vi "Process.vi"(8 "error in":errorcluster, 11 "XYStage.KIM101":refnum<class "XYStage.KIM101.lvclass">) -> (0 "error out":errorcluster, 3 "XYStage.KIM101 out":refnum<class "XYStage.KIM101.lvclass">)   [LabVIEW 2017, in "XYStage.KIM101.lvclass"]
doc: "---------------------------------------------------------------\nJKI State Machine Objects™\nhttp://jki.net/state-machine-objects/\nCopyright (C) 2005-2015, JKI <info@jki.net>\nALL RIGHTS RESERVEDJKI State Machine Objects (SMO) 1.0.0.5\nJKI - JKI\nCopyright (c) 2016, JKI"
uses:
  XYStage.KIM101.lvclass
  D:/Program Files (x86)/National Instruments/LabVIEW 2017/vi.lib/JKI/JKI SMO/SMO/SMO.lvclass
  D:/upwork/Laser Measurement Tool/Laser/project/Subsystems/XYStage/XYStage.lvclass
  D:/upwork/Laser Measurement Tool/Laser/project/Subsystems/Device/Device.lvclass
  <vilib>/JKI/JKI SMO/SMO/Typedefs/Parent Call--Enum.ctl
  XYStage/Typedefs/ProtectedEvents--XYStage.StatusUpdated.ctl
  XYStage/Typedefs/XYStage.Axis--Enum.ctl
  XYStage/Typedefs/XYStage.DeviceStatus--Enum.ctl
  Typedefs/InertialMotorStatus--Cluster.ctl
  XYStage/Typedefs/Coordinates--Cluster.ctl
  XYStage/Typedefs/Coordinates.Units--Cluster.ctl
  XYStage/Typedefs/Coordinates.Counts--Cluster.ctl
  Typedefs/Wait--Cluster.ctl
  Typedefs/Move Result--Cluster.ctl
  XYStage/Typedefs/ProtectedEvents--XYStage.MoveResultReported.ctl
  StatusUpdate Callback.vi
  XYStage/XYStage.lvclass
  <vilib>/JKI/JKI SMO/SMO/SMO.lvclass
  Device/Device.lvclass
  D:/upwork/Laser Measurement Tool/Laser/project/data/Thorlabs.MotionControl.KCube.InertialMotorCLI.dll
  data/Thorlabs.MotionControl.KCube.InertialMotorCLI.dll
panel:
  # "XYStage.KIM101\nProcess.vi"
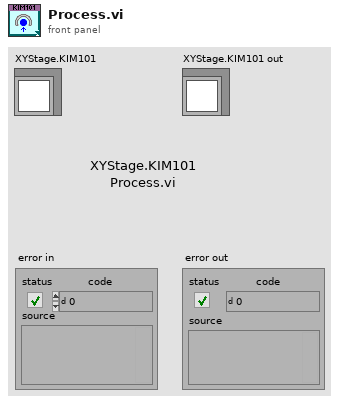
[diagram p1: front panel]
types:
  T1 = typedef "SMO.lvclass/Parent Call--Enum.ctl" = enum16{"Allows parent to run", "Does not request parent to run"}
  T2 = enum32{"invalid app kind", "Development System", "Run Time System", "Student Edition", "Embedded LabVIEW", "Evaluation", "Custom"}
  T3 = enum32{"Invalid", "Standard", "Closed", "Hidden", "Minimized", "Maximized"}
  T4 = typedef "XYStage.lvclass/XYStage.Axis--Enum.ctl" = enum16{"X Axis", "Y Axis", "Undefined"}
  T5 = typedef "Device.lvclass/PublicEvents--Device.Initialized.ctl" = bool
  T6 = typedef "XYStage.lvclass/Coordinates--Cluster.ctl" = cluster{"Units":T7, "Counts":T8}
  T7 = typedef "XYStage.lvclass/Coordinates.Units--Cluster.ctl" = cluster{"X":dbl, "Y":dbl}
  T8 = typedef "XYStage.lvclass/Coordinates.Counts--Cluster.ctl" = cluster{"X":i32, "Y":i32}
  T9 = typedef "XYStage.KIM101.lvclass/Wait--Cluster.ctl" = cluster{"Axis":T4, "In Wait?":bool, "Position":i32, "Next Steps":string, "Result":bool}
  T10 = typedef "XYStage.lvclass/ProtectedEvents--XYStage.StatusUpdated.ctl" = cluster{"Axis":T4, "Position":i32, "IsEnabled":bool, "IsError":bool, "IsMoving":bool, "Status":T11}
  T11 = typedef "XYStage.lvclass/XYStage.DeviceStatus--Enum.ctl" = u32
  T12 = typedef "XYStage.KIM101.lvclass/Move Result--Cluster.ctl" = cluster{"X axis need to move?":bool, "X axis move result":bool, "Y axis need to move?":bool, "Y axis move result":bool}
  T13 = cluster{"Core":cluster{"Current VI Reference":refnum<vi>, "Close Panel on Exit?":bool, "error":errorcluster}, "Self Reference":refnum<class "XYStage.KIM101.lvclass">, "Status Update Event":refnum<user-event>, "Initialized":bool, "Wait Timeout, ms":i32, "Target":T6, "Current":T6, "Wait":T9, "StatusUpdated":T10, "Move Result":T12}
  T14 = cluster{"Current VI Reference":refnum<vi>, "Close Panel on Exit?":bool, "error":errorcluster}
  T15 = typedef "XYStage.KIM101.lvclass/InertialMotorStatus--Cluster.ctl" = cluster{"Channel":i32, "IsEnabled":bool, "IsError":bool, "IsMoving":bool, "Position":i32, "Status":u32}
  T16 = typedef "SMO.lvclass/Protected Events.ctl" = cluster{"StopProcesses":refnum<user-event>, "AbortProcesses":refnum<user-event>, "Config Changed":refnum<user-event>, "Dependency":refnum<user-event>}
  T17 = cluster{"Event Registration Refnum":refnum<event-registration>, "Device Public Events":refnum<event-registration>, "Event Registration Refnum":refnum<event-registration>, "XYStage.KIM101 Private Events":refnum<event-registration>}
  T18 = typedef "XYStage.lvclass/ProtectedEvents--XYStage.MoveResultReported.ctl" = cluster{"Result":bool, "Coordinates":T6}
  T19 = typedef "XYStage.KIM101.lvclass/Resource--Cluster.ctl" = cluster{"KCubeInertialMotorControl":refnum<k24>, "Device":refnum<k24>, "X Axis Channel":i32, "Y Axis Channel":i32}
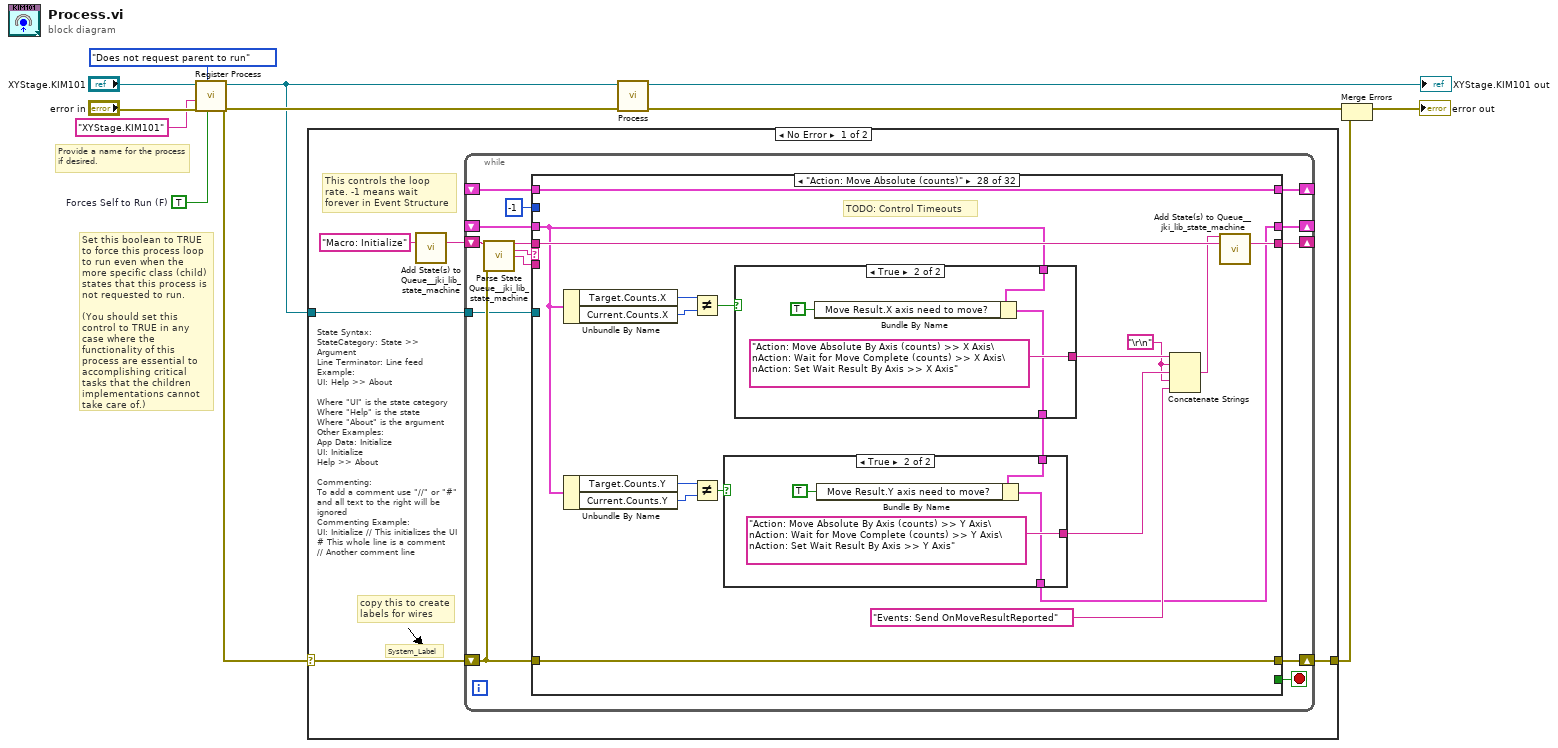
[diagram p0: block diagram]
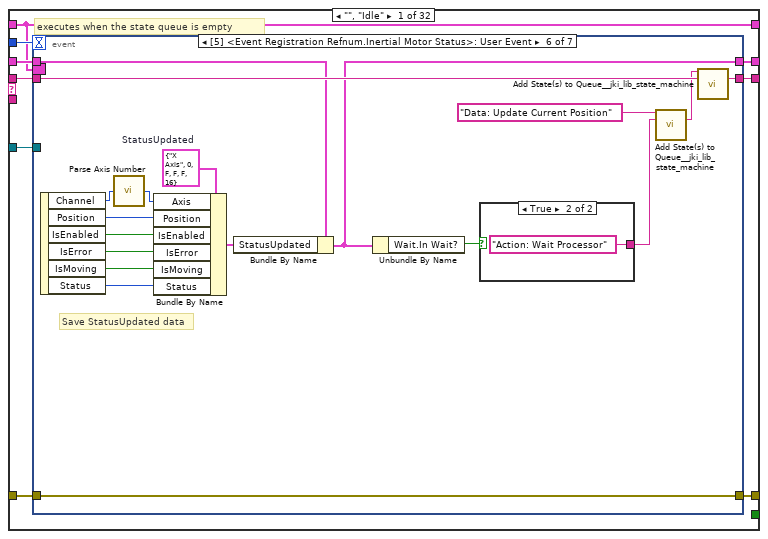
[diagram p2: hidden frame]
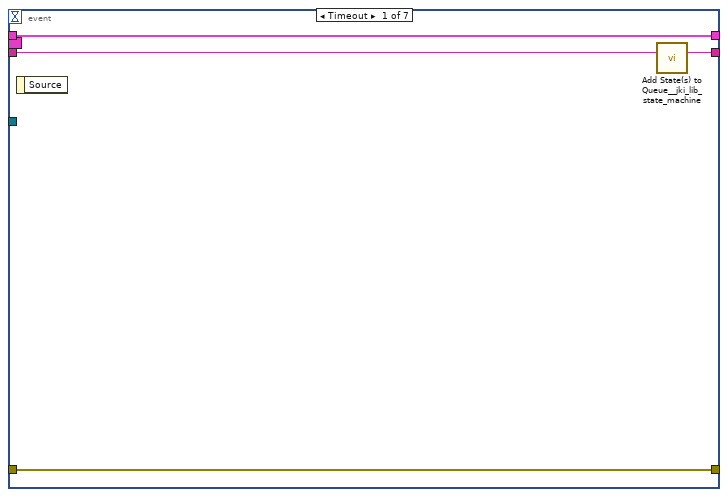
[diagram p3: hidden frame]
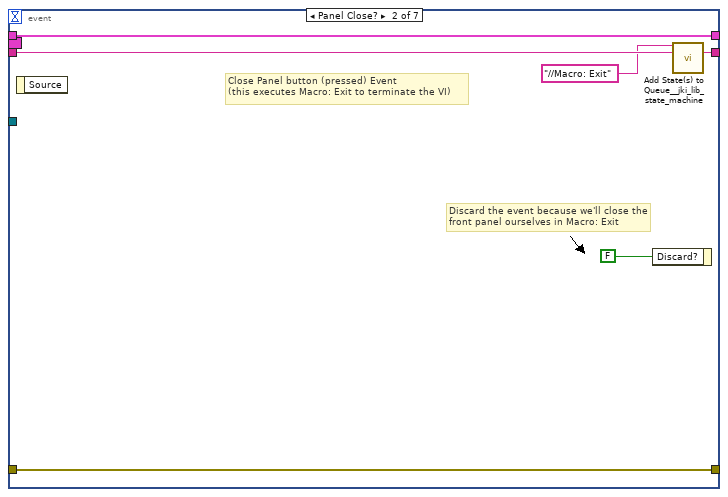
[diagram p4: hidden frame]
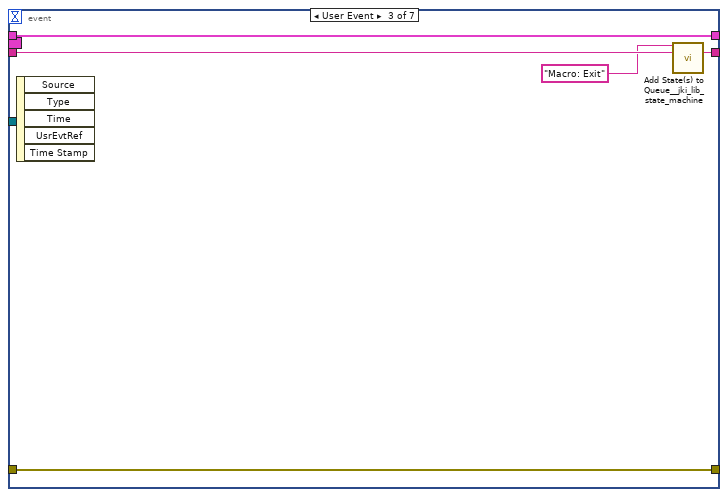
[diagram p5: hidden frame]
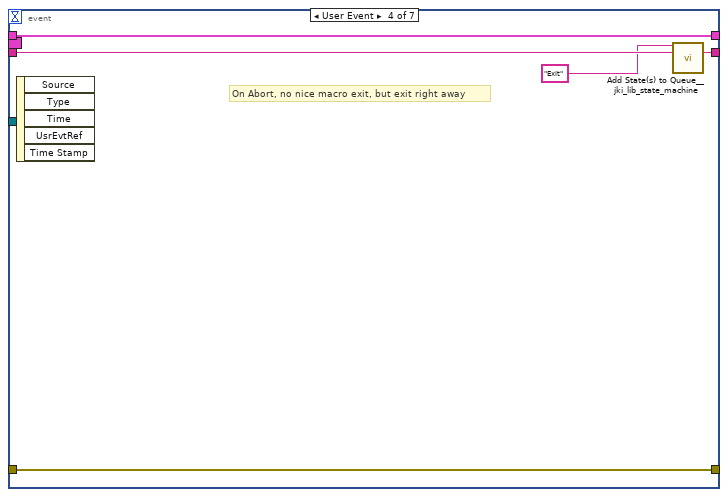
[diagram p6: hidden frame]
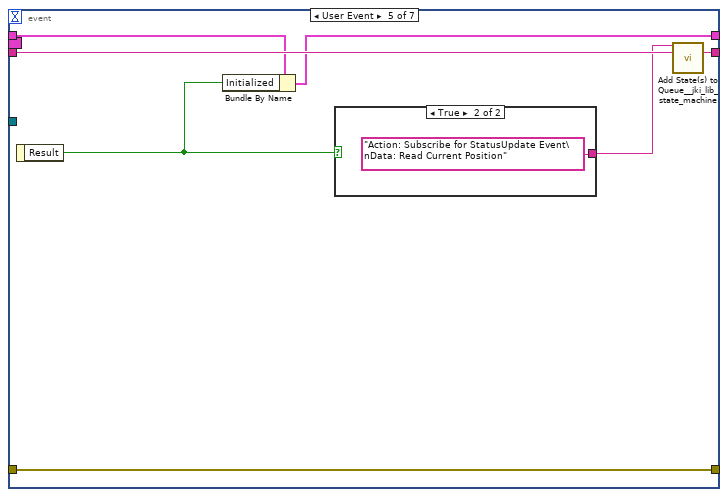
[diagram p7: hidden frame]
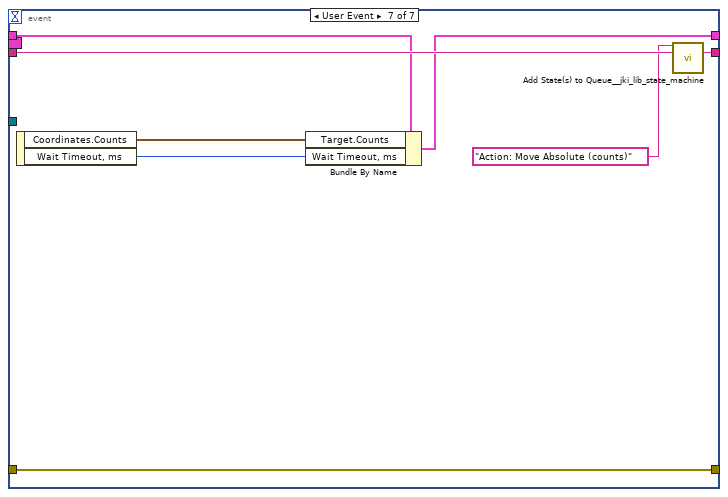
[diagram p10: hidden frame]
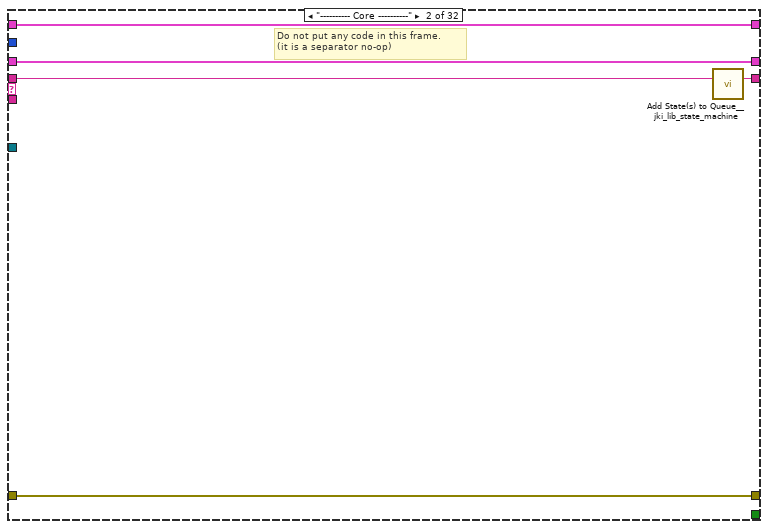
[diagram p11: hidden frame]
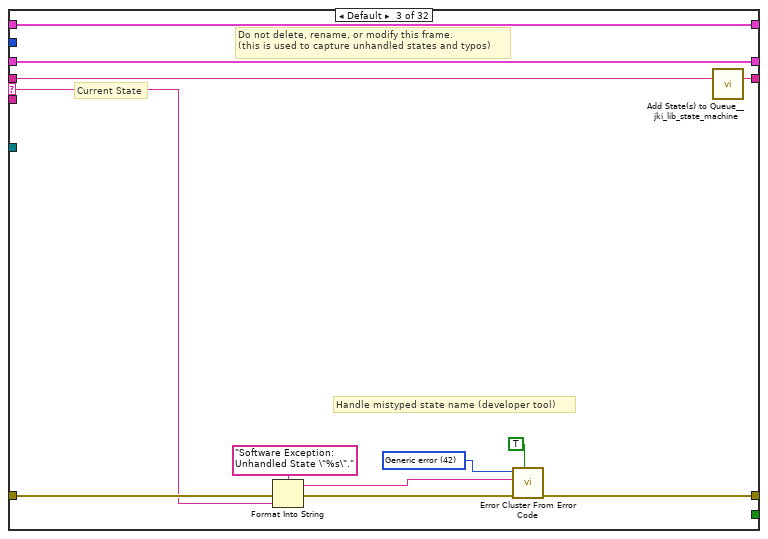
[diagram p12: hidden frame]
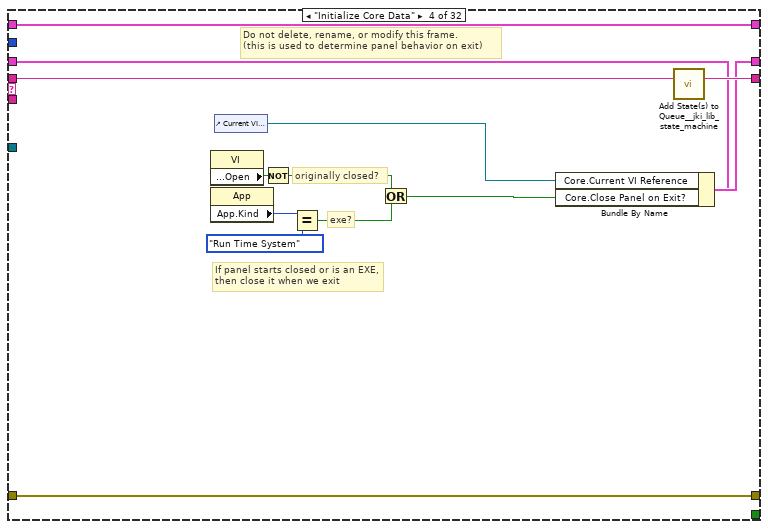
[diagram p13: hidden frame]
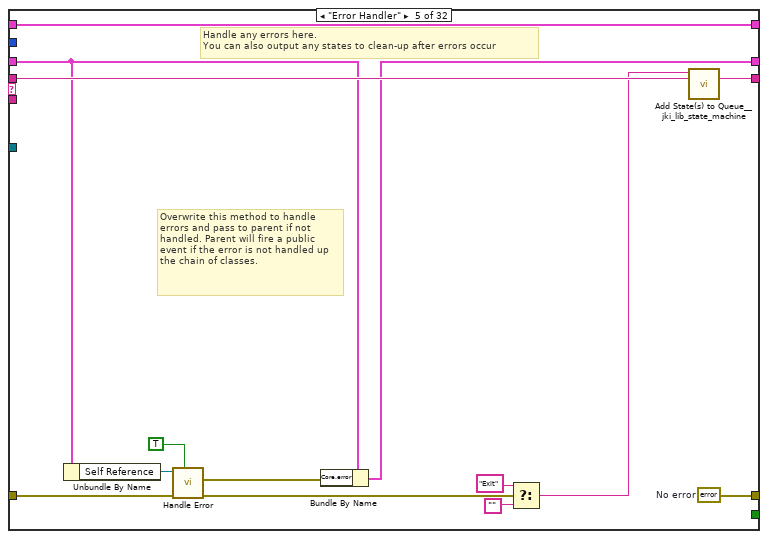
[diagram p14: hidden frame]
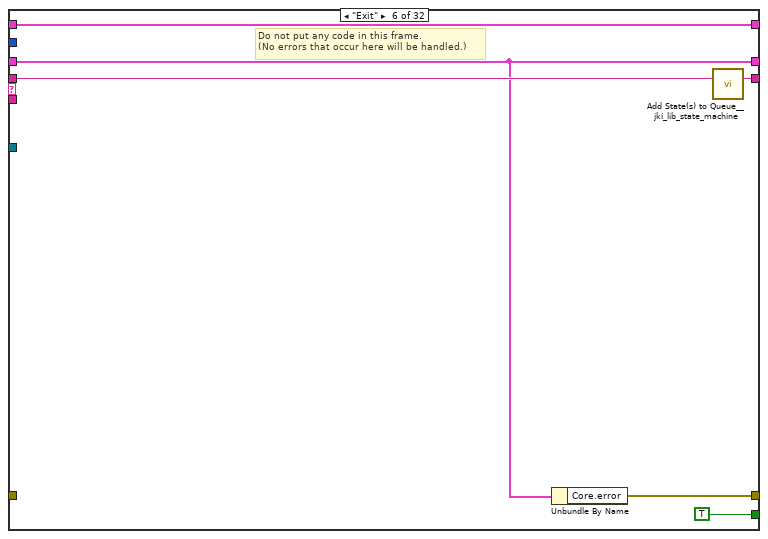
[diagram p15: hidden frame]
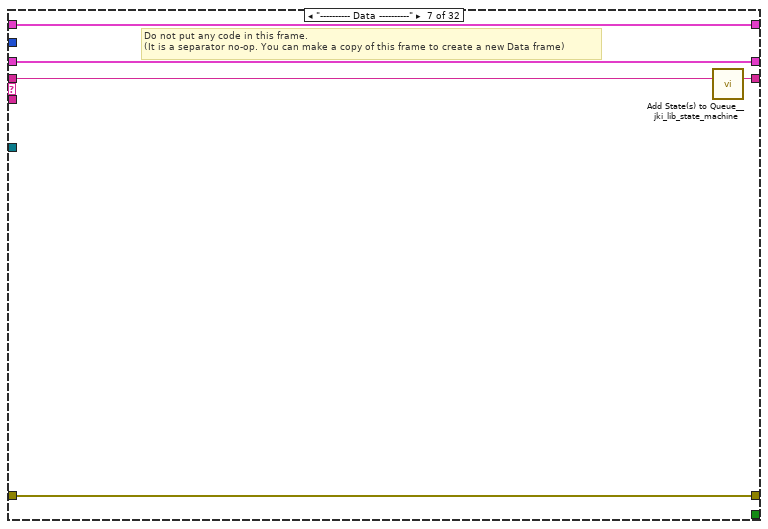
[diagram p16: hidden frame]
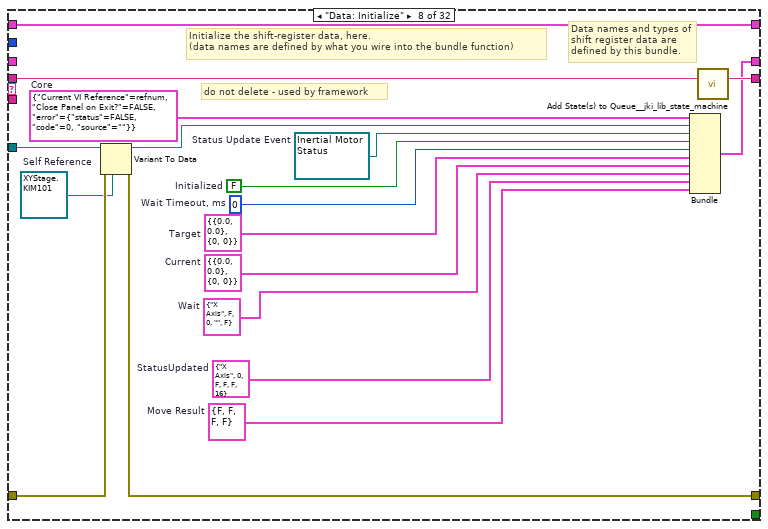
[diagram p17: hidden frame]
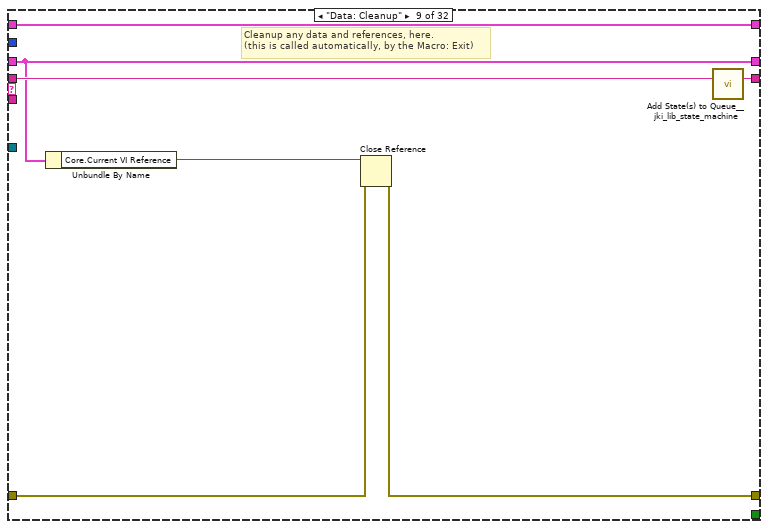
[diagram p18: hidden frame]
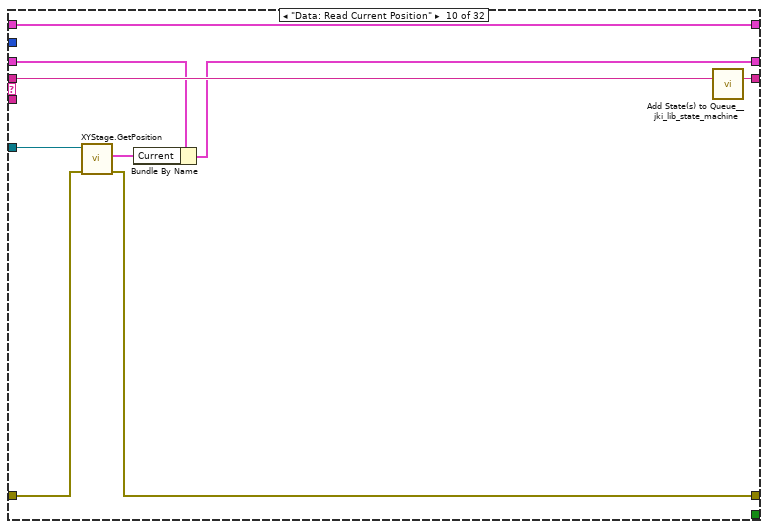
[diagram p19: hidden frame]
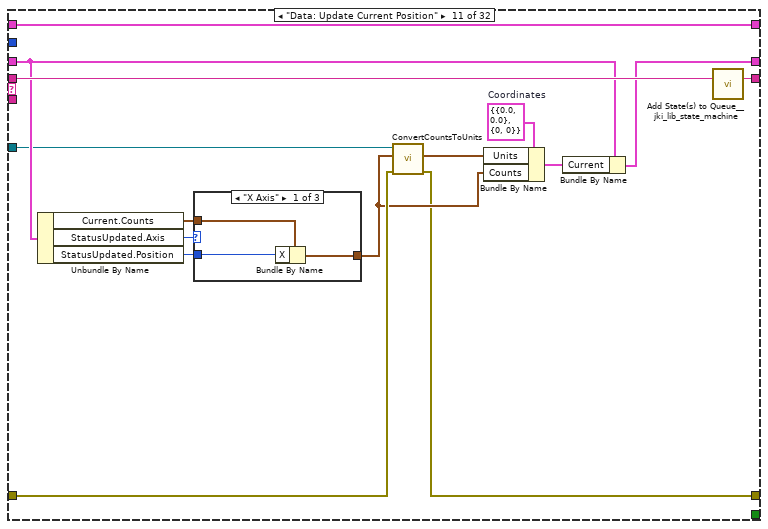
[diagram p20: hidden frame]
diagram:
  w2 = TRUE  # Forces Self to Run (F)
  # "Provide a name for the process\nif desired."
  # "Set this boolean to TRUE to force this process loop to run even when the more specific class (child) states that this process is not requested to run.\n\n(You should set this control to TRUE in any case where the functionality of this process are essential to accomplishing critical tasks that the children implementations cannot take care of.)"
  n1 = call <vilib>:"Register Process.vi"("Forces Self to Run (F)"=w2, "Parent Call"=Parent_Call--Enum."Does not request parent to run", "error in (no error)"="error in", "Process Name (optional)"="XYStage.KIM101", "SMO"="XYStage.KIM101") -> ("error out"=w8:errorcluster, "SMO out"=w7:refnum<class "XYStage.KIM101.lvclass">)  [unwired: 5 in]
  n2 = case shown="No Error" w8 {
    selector: w8 -> [w13 w496]
    tunnel: w7 -> [w14 _]
    tunnel: [w12 w496] -> w4
    frame No Error {
      # "State Syntax:\nStateCategory: State >> Argument\nLine Terminator: Line feed\nExample:\nUI: Help >> About\n\nWhere \"UI\" is the state category\nWhere \"Help\" is the state\nWhere \"About\" is the argument\nOther Examples:\nApp Data: Initialize\nUI: Initialize\nHelp >> About\n\nCommenting:\nTo add a comment use \"//\" or \"#\" and all text to the right will be ignored\nCommenting Example:\nUI: Initialize // This initializes the UI\n# This whole line is a comment\n// Another comment line"
      # "copy this to create labels for wires"
      # "This controls the loop rate. -1 means wait forever in Event Structure"
      # "System_Label"
      n3 = call <vilib>:"Add State(s) to Queue__jki_lib_state_machine.vi"("State(s) in (\"\")"="Macro: Initialize") -> ("States Out"=w16:string)  [unwired: 14 in]
      n4 = while {
        shift-right: [w23] -> _
        shift-left: _ -> [w22]
        shift-right: [w26] -> w12
        shift-left: w13 -> [w20]
        shift-right: [w25] -> _
        shift-left: w16 -> [w27]
        tunnel: w14 -> [w19]
        shift-right: [w18] -> _
        shift-left: _ -> [w17]
        stop <- w24 stop-if-true
        n5 = call <vilib>:"Parse State Queue__jki_lib_state_machine.vi"("State Queue"=w27, "Error In (no error)"=w20) -> ("Remaining States"=w29:string, "Current State"=w30:string, "Arguments"=w28:string)  [unwired: 11 in]
        n6 = case shown="\"Events: Send OnMoveResultReported\"" w30 {
          selector: w30 -> [_ _ w101 _ _ _ _ _ _ _ _ _ _ _ _ _ _ _ _ _ _ _ _ _ _ _ _ _ _ _ _ _]
          tunnel: w29 -> [w39 w99 w105 w124 w138 w144 w149 w167 w174 w183 w198 w210 w215 w222 w238 w270 w279 w293 w298 w309 w314 w337 w343 w351 w368 w377 w389 w407 w431 w438 w466 w488]
          tunnel: w28 -> [_ _ _ _ _ _ _ _ _ _ _ _ _ w216 w232 _ _ _ _ _ _ _ _ _ _ _ _ _ w425 w444 _ w484]
          tunnel: w22 -> [w37 w96 w103 w115 w127 w140 w146 _ w169 w178 w194 w207 w213 w220 w234 w267 w275 w284 w295 w306 w311 w323 w341 w348 w365 w375 w382 w392 w424 w443 w457 w482]
          tunnel: [w36 w97 w107 w121 w129 w139 w147 w163 w170 w175 w184 w208 w212 w217 w235 w268 w277 w291 w296 w300 w312 w331 w339 w344 w362 w373 w378 w404 w426 w445 w463 w485] -> w26
          tunnel: w20 -> [w35 w97 w106 w121 w134 _ w147 w164 w171 w176 w189 w208 w212 w218 w236 w268 w277 w291 w296 w301 w312 w333 w339 w345 w363 w373 w380 w404 w427 w445 w463 w485]
          tunnel: [w38 w98 w104 w123 w137 w143 w148 w166 w173 w182 w197 w209 w214 w221 w237 w269 w278 w292 w297 w308 w313 w336 w342 w350 w367 w376 w388 w406 w430 w447 w465 w487] -> w25
          tunnel: [_ _ _ _ _ TRUE _ _ _ _ _ _ _ _ _ _ _ _ _ _ _ _ _ _ _ _ _ _ _ _ _ _] -> w24
          tunnel: [w34 w96 w103 w122 w126 w140 w146 w165 w169 w177 w195 w207 w213 w220 w234 w267 w275 w284 w295 w306 w311 w321 w341 w348 w365 w375 w382 w390 w424 w442 w456 w481] -> w23
          tunnel: -1 ("Timeout") -> [w33 _ _ _ _ _ _ _ _ _ _ _ _ _ _ _ _ _ _ _ _ _ _ _ _ _ _ _ _ _ _ _]
          tunnel: w19 -> [w31 _ _ _ _ _ _ w161 _ w180 w190 _ _ _ _ _ _ _ _ _ _ _ _ w347 w364 _ w387 _ w428 _ _ _]
          tunnel: [w32 w95 w100 w112 w136 w141 w145 w159 w168 w181 w196 w206 w211 w219 w231 w266 w276 w285 w294 w307 w310 w329 w340 w349 w366 w374 w383 w405 w429 w446 w464 w486] -> w18
          tunnel: w17 -> [w32 w95 w100 w112 w136 w141 w145 w159 w168 w181 w196 w206 w211 w219 w231 w266 w276 w285 w294 w307 w310 _ w340 w349 w366 w374 w383 w405 w429 w446 w464 w486]
          frame "", "Idle" {
            # "executes when the state queue is empty"
            n7 = event shown="[5] <Event Registration Refnum.Inertial Motor Status>: User Event" {
              selector: w32 -> [_ _ _ _ _ _ _]
              dyn-events: _ -> [_ _ _ _ _ _ _]
              timeout: w33 -> [_ _ _ _ _ _ _]
              tunnel: w39 -> [w43 w49 w54 w59 w66 w85 w94]
              tunnel: [w42 w48 w53 w58 w65 w84 w93] -> w38
              tunnel: w37 -> [w40 w46 w51 w56 w62 w73 w90]
              tunnel: [w41 w47 w52 w57 w64 w78 w92] -> w36
              tunnel: w35 -> [w41 w47 w52 w57 w64 w78 w92]
              tunnel: [w40 w46 w51 w56 w60 w72 w89] -> w34
              tunnel: w31 -> [_ _ _ _ _ _ _]
              event Timeout {
                n8 = event-data() -> ()  [unwired: 1 in, 1 out]
                n9 = call <vilib>:"Add State(s) to Queue__jki_lib_state_machine.vi"("State(s) in (\"\")"=w43) -> ("States Out"=w42:string)  [unwired: 14 in]
              }
              event Panel Close? {
                # "Discard the event because we'll close the front panel ourselves in Macro: Exit"
                # "Close Panel button (pressed) Event\n(this executes Macro: Exit to terminate the VI)"
                n10 = event-data() -> ()  [unwired: 1 in, 1 out]
                n11 = event-data("Discard?"=FALSE) -> ()  [unwired: 1 in, 1 out]
                n12 = call <vilib>:"Add State(s) to Queue__jki_lib_state_machine.vi"("State(s) in Front (\"\")"="//Macro: Exit", "State(s) in (\"\")"=w49) -> ("States Out"=w48:string)  [unwired: 13 in]
              }
              event User Event {
                n13 = event-data() -> ()  [unwired: 1 in, 5 out]
                n14 = call <vilib>:"Add State(s) to Queue__jki_lib_state_machine.vi"("State(s) in Front (\"\")"="Macro: Exit", "State(s) in (\"\")"=w54) -> ("States Out"=w53:string)  [unwired: 13 in]
              }
              event User Event {
                # "On Abort, no nice macro exit, but exit right away"
                n15 = event-data() -> ()  [unwired: 1 in, 5 out]
                n16 = call <vilib>:"Add State(s) to Queue__jki_lib_state_machine.vi"("State(s) in Front (\"\")"="Exit", "State(s) in (\"\")"=w59) -> ("States Out"=w58:string)  [unwired: 13 in]
              }
              event User Event {
                n17 = event-data() -> ("Result"=w61:T5)  [unwired: 1 in]
                n18 = Bundle By Name(cluster=w62, "Initialized"=w61) -> (w60:T13)
                n19 = case shown="True" w61 {
                  tunnel: [_ "Action: Subscribe for StatusUpdate Event\nData: Read Current Position"] -> w63
                  frame False {
                  }
                  frame True {
                  }
                }
                n20 = call <vilib>:"Add State(s) to Queue__jki_lib_state_machine.vi"("State(s) in Front (\"\")"=w63, "State(s) in (\"\")"=w66) -> ("States Out"=w65:string)  [unwired: 13 in]
              }
              event User Event {
                w83 = T10 {"Axis"=enum."X Axis", "Position"=0, "IsEnabled"=FALSE, "IsError"=FALSE, "IsMoving"=FALSE, "Status"=16}  # StatusUpdated
                # "Save StatusUpdated data"
                n21 = event-data() -> ("Channel"=w77:i32, "Position"=w74:i32, "IsEnabled"=w82:bool, "IsError"=w81:bool, "IsMoving"=w80:bool, "Status"=w79:u32)  [unwired: 1 in]
                n22 = call "Parse Axis Number.vi"("Channel"=w77) -> ("Axis"=w75:T4)
                n23 = Bundle By Name(cluster=w83, "Axis"=w75, "Position"=w74, "IsEnabled"=w82, "IsError"=w81, "IsMoving"=w80, "Status"=w79) -> (w76:T10)
                n24 = Bundle By Name(cluster=w73, "StatusUpdated"=w76) -> (w72:T13)
                n25 = Unbundle By Name(w72) -> ("Wait.In Wait?"=w71:bool)
                n26 = case shown="True" w71 {
                  tunnel: [_ "Action: Wait Processor"] -> w68
                  frame False {
                  }
                  frame True {
                  }
                }
                n27 = call <vilib>:"Add State(s) to Queue__jki_lib_state_machine.vi"("State(s) in Front (\"\")"="Data: Update Current Position" ("State(s) in Front (\"\")"), "State(s) in (\"\")"=w68) -> ("States Out"=w69:string)  [unwired: 13 in]
                n28 = call <vilib>:"Add State(s) to Queue__jki_lib_state_machine.vi"("State(s) in Front (\"\")"=w69, "State(s) in (\"\")"=w85) -> ("States Out"=w84:string)  [unwired: 13 in]
              }
              event User Event {
                n29 = event-data() -> ("Coordinates.Counts"=w91:T8, "Wait Timeout, ms"=w87:i32)  [unwired: 1 in]
                n30 = Bundle By Name(cluster=w90, "Target.Counts"=w91, "Wait Timeout, ms"=w87) -> (w89:T13)
                n31 = call <vilib>:"Add State(s) to Queue__jki_lib_state_machine.vi"("State(s) in Front (\"\")"="Action: Move Absolute (counts)" ("State(s) in Front (\"\")"), "State(s) in (\"\")"=w94) -> ("States Out"=w93:string)  [unwired: 13 in]
              }
            }
          }
          frame "---------- Core ----------" {
            # "Do not put any code in this frame.\n(it is a separator no-op)"
            n32 = call <vilib>:"Add State(s) to Queue__jki_lib_state_machine.vi"("State(s) in (\"\")"=w99) -> ("States Out"=w98:string)  [unwired: 14 in]
          }
          frame Default {
            w110 = 42 items=["No error", "Argument error", "Memory is full", "Out of zone", "End of file", "File already open", "Generic file I/O error", "File not found", "File permission error", "Disk is full", "Duplicate path", "Too many files open", "System feature not enabled", "Resource file not found", "Cannot add resource", "Resource not found", "Image not found", "Image memory error", "Pen does not exist", "Config type invalid", "Config token not found", "Config parse error", "Config memory error", "Bad external code format", "Bad external code offset", "External code not present", "Null window", "Destroy window error", "Null menu", "Print aborted", "Bad print record", "Print driver error", "Windows error during printing", "Memory error during printing", "Print dialog error", "Generic print error", "Invalid device refnum", "Device not found", "Device parameter error", "Device unit error", "Cannot open device", "Device call aborted", "Generic error", "Cancelled by user", "Object ID too low", "Object ID too high", "Object not in heap", "Unknown heap", "Unknown object (invalid DefProc)", "Unknown object (DefProc not in table)", "Message out of range", "Invalid (null) method", "Unknown message", "Manager call not supported", "Bad address", "Network operation in progress", "Network operation timed out", "Connection is busy", "Network attribute not supported", "Network error", "Address in use", "System out of memory", "Connection aborted", "Connection refused", "Not connected", "Already connected", "Connection closed", "Initialization error (interapplication manager)", "Bad occurrence", "Wait on unbound occurrence handler", "Occurrence queue overflow", "Datalog type conflict", "Unused", "Unrecognized type (interapplication manager)", "Memory corrupt", "Failed to make temporary DLL", "Old CIN version", "Drag socket not found", "Failed to load drop-object", "Failed to register OLE object", "Failed to release OLE object", "Format specifier type mismatch", "Unknown format specifier", "Too few format specifiers", "Too many format specifiers", "Scan failed", "Newer CIN version", "Error converting to variant", "Runtime menu error", "Password tampered", "Variant attribute not found", "Incompatible variant data type", "Event data is not available", "Event Store is not present", "Occurrence is not found", "Event Queue is not created", "Event info is not available", "Refnum passed is NULL", "Error retrieving Class GUID", "Error retrieving CoClass GUID", "Error retrieving TypeLib GUID.", "Bad built application magic bytes.", "Specific driver is different from the specific driver associated with the Logical Name.", "There is no session opened to the class driver.", "Max Error", "MAX - Error with config objects", "MAX - Error loading configuration", "MAX - Group not supported"]
            # "Current State"
            # "Do not delete, rename, or modify this frame.\n(this is used to capture unhandled states and typos)"
            # "Handle mistyped state name (developer tool)"
            n33 = Format Into String(format string="Software Exception: Unhandled State \"%s\"." ("message"), error in=w106, w101) -> (resulting string=w109:string, error out=w108:errorcluster)  [unwired: 1 in]
            n34 = call <vilib>:"Error Cluster From Error Code.vi"("show call chain? (False)"=TRUE, "error in (no error)"=w108, "error message (\"\")"=w109, "error code (0)"=w110) -> ("error out"=w107:errorcluster)  [unwired: 5 in]
            n35 = call <vilib>:"Add State(s) to Queue__jki_lib_state_machine.vi"("State(s) in (\"\")"=w105) -> ("States Out"=w104:string)  [unwired: 14 in]
          }
          frame "Initialize Core Data" {
            # "Do not delete, rename, or modify this frame.\n(this is used to determine panel behavior on exit)"
            # "originally closed?"
            # "exe?"
            # "If panel starts closed or is an EXE, then close it when we exit"
            n36 = property class="VI"() -> ("Front Panel.Open"=w120:bool)  [unwired: 2 in, 2 out]
            n37 = property class="App"() -> ("App.Kind"=w119:T2)  [unwired: 2 in, 2 out]
            n38 = control-ref of="Current VI Reference"() -> (w113:refnum<vi>)
            n39 = Not(x=w120) -> (.not. x?=w117:bool)
            n40 = Equal?(x=w119, y=T2."Run Time System" ("Application:Kind")) -> (x = y?=w116:bool)
            n41 = Or(x=w117, y=w116) -> (x .or. y?=w114:bool)
            n42 = Bundle By Name(cluster=w115, "Core.Current VI Reference"=w113, "Core.Close Panel on Exit?"=w114) -> (w122:T13)
            n43 = call <vilib>:"Add State(s) to Queue__jki_lib_state_machine.vi"("State(s) in (\"\")"=w124) -> ("States Out"=w123:string)  [unwired: 14 in]
          }
          frame "Error Handler" {
            w129 = errorcluster {"status"=FALSE, "code"=0, "source"=""}  # No error
            # "Overwrite this method to handle errors and pass to parent if not handled. Parent will fire a public event if the error is not handled up the chain of classes."
            # "Handle any errors here.\nYou can also output any states to clean-up after errors occur"
            n44 = Unbundle By Name(w127) -> ("Self Reference"=w135:refnum<class "XYStage.KIM101.lvclass">)
            n45 = call-dynamic "Handle Error.vi"("Stop on Unhandled Error (T)"=TRUE, "error in"=w134, "SMO"=w135) -> ("handling error"=w130:errorcluster, "Unhandled error"=w128:errorcluster)  [unwired: 6 in, 1 out]
            n46 = Bundle By Name(cluster=w127, "Core.error"=w128) -> (w126:T13)
            n47 = Select(t="Exit", s=w130, f="") -> (s? t:f=w131:string)
            n48 = call <vilib>:"Add State(s) to Queue__jki_lib_state_machine.vi"("State(s) in Front (\"\")"=w131, "State(s) in (\"\")"=w138) -> ("States Out"=w137:string)  [unwired: 13 in]
          }
          frame "Exit" {
            # "Do not put any code in this frame.\n(No errors that occur here will be handled.)"
            n49 = Unbundle By Name(w140) -> ("Core.error"=w139:errorcluster)
            n50 = call <vilib>:"Add State(s) to Queue__jki_lib_state_machine.vi"("State(s) in (\"\")"=w144) -> ("States Out"=w143:string)  [unwired: 14 in]
          }
          frame "---------- Data ----------" {
            # "Do not put any code in this frame.\n(It is a separator no-op. You can make a copy of this frame to create a new Data frame)"
            n51 = call <vilib>:"Add State(s) to Queue__jki_lib_state_machine.vi"("State(s) in (\"\")"=w149) -> ("States Out"=w148:string)  [unwired: 14 in]
          }
          frame "Data: Initialize" {
            w150 = T12 {"X axis need to move?"=FALSE, "X axis move result"=FALSE, "Y axis need to move?"=FALSE, "Y axis move result"=FALSE}  # Move Result
            w151 = T9 {"Axis"=enum."X Axis", "In Wait?"=FALSE, "Position"=0, "Next Steps"="", "Result"=FALSE}  # Wait
            w152 = T10 {"Axis"=enum."X Axis", "Position"=0, "IsEnabled"=FALSE, "IsError"=FALSE, "IsMoving"=FALSE, "Status"=16}  # StatusUpdated
            w153 = T6 {"Units"={"X"=0.0, "Y"=0.0}, "Counts"={"X"=0, "Y"=0}}  # Current
            w156 = 0  # Wait Timeout, ms
            w154 = T6 {"Units"={"X"=0.0, "Y"=0.0}, "Counts"={"X"=0, "Y"=0}}  # Target
            w157 = FALSE  # Initialized
            w155 = refnum<user-event> refnum  # Status Update Event
            w158 = T14 {"Current VI Reference"=refnum, "Close Panel on Exit?"=FALSE, "error"={"status"=FALSE, "code"=0, "source"=""}}  # Core
            w162 = refnum<class "XYStage.KIM101.lvclass"> refnum  # Self Reference
            # "do not delete - used by framework"
            # "Data names and types of shift register data are defined by this bundle."
            # "Initialize the shift-register data, here.\n(data names are defined by what you wire into the bundle function)"
            n52 = Variant To Data(error in=w164, type=w162, Variant=w161) -> (data=w160:refnum<class "XYStage.KIM101.lvclass">, error out=w163:errorcluster)
            n53 = Bundle("Core"=w158, "Self Reference"=w160, "Status Update Event"=w155, "Initialized"=w157, "Wait Timeout, ms"=w156, "Target"=w154, "Current"=w153, "Wait"=w151, "StatusUpdated"=w152, "Move Result"=w150) -> (w165:T13)  [unwired: 1 in]
            n54 = call <vilib>:"Add State(s) to Queue__jki_lib_state_machine.vi"("State(s) in (\"\")"=w167) -> ("States Out"=w166:string)  [unwired: 14 in]
          }
          frame "Data: Cleanup" {
            # "Cleanup any data and references, here.\n(this is called automatically, by the Macro: Exit)"
            n55 = Unbundle By Name(w169) -> ("Core.Current VI Reference"=w172:refnum<vi>)
            n56 = Close Reference(reference=w172, error in (no error)=w171) -> (error out=w170:errorcluster)
            n57 = call <vilib>:"Add State(s) to Queue__jki_lib_state_machine.vi"("State(s) in (\"\")"=w174) -> ("States Out"=w173:string)  [unwired: 14 in]
          }
          frame "Data: Read Current Position" {
            n58 = call-dynamic "XYStage.GetPosition.vi"("error in (no error)"=w176, "XYStage.KIM101 in"=w180) -> ("error out"=w175:errorcluster, "Coordinates"=w179:T6)  [unwired: 7 in, 1 out]
            n59 = Bundle By Name(cluster=w178, "Current"=w179) -> (w177:T13)
            n60 = call <vilib>:"Add State(s) to Queue__jki_lib_state_machine.vi"("State(s) in (\"\")"=w183) -> ("States Out"=w182:string)  [unwired: 14 in]
          }
          frame "Data: Update Current Position" {
            w188 = T6 {"Units"={"X"=0.0, "Y"=0.0}, "Counts"={"X"=0, "Y"=0}}  # Coordinates
            n61 = Unbundle By Name(w194) -> ("Current.Counts"=w192:T8, "StatusUpdated.Axis"=w193:T4, "StatusUpdated.Position"=w191:i32)
            n62 = case shown="\"X Axis\"" w193 {
              tunnel: w192 -> [w201 w204 w205]
              tunnel: w191 -> [w200 w202 _]
              tunnel: [w199 w203 w205] -> w186
              frame "X Axis" {
                n63 = Bundle By Name(cluster=w201, "X"=w200) -> (w199:T8)
              }
              frame "Y Axis" {
                n64 = Bundle By Name(cluster=w204, "Y"=w202) -> (w203:T8)
              }
              frame "Undefined", Default {
              }
            }
            n65 = call "ConvertCountsToUnits.vi"("error in (no error)"=w189, "Coordinates.Counts"=w186, "XYStage in"=w190) -> ("error out"=w184:errorcluster, "Coordinates.Units"=w187:T7)  [unwired: 6 in, 1 out]
            n66 = Bundle By Name(cluster=w188, "Units"=w187, "Counts"=w186) -> (w185:T6)
            n67 = Bundle By Name(cluster=w194, "Current"=w185) -> (w195:T13)
            n68 = call <vilib>:"Add State(s) to Queue__jki_lib_state_machine.vi"("State(s) in (\"\")"=w198) -> ("States Out"=w197:string)  [unwired: 14 in]
          }
          frame "---------- UI ----------" {
            # "Do not put any code in this frame.\n(It is a separator no-op. You can make a copy of this frame to create a new UI frame)"
            n69 = call <vilib>:"Add State(s) to Queue__jki_lib_state_machine.vi"("State(s) in (\"\")"=w210) -> ("States Out"=w209:string)  [unwired: 14 in]
          }
          frame "UI: Initialize" {
            # "Initialize the User Interface, here.\n(this is called automatically, by the Macro: Init)"
            n70 = call <vilib>:"Add State(s) to Queue__jki_lib_state_machine.vi"("State(s) in (\"\")"=w215) -> ("States Out"=w214:string)  [unwired: 14 in]
          }
          frame "UI: Cursor Set" {
            # "Argument"
            # "Initialize the User Interface, here.\n(this is called automatically, by the Macro: Init)"
            n71 = disable-structure shown="Default" {
              disable-tunnel: w218 -> [w223 w226]
              disable-tunnel: [w223 w225] -> w217
              disable-tunnel: w216 -> [_ w224]
              frame condition #0 {
              }
              frame condition #1 (active) {
                n72 = case shown="\"Idle\", Default" w224 {
                  tunnel: w226 -> [w228 w230]
                  tunnel: [w227 w229] -> w225
                  frame "Idle", Default {
                    n73 = call <vilib>:"Unset Busy.vi"("error in (no error)"=w228) -> ("error out"=w227:errorcluster)  [unwired: 10 in]
                  }
                  frame "Busy" {
                    n74 = call <vilib>:"Set Busy.vi"("error in (no error)"=w230) -> ("error out"=w229:errorcluster)  [unwired: 9 in, 1 out]
                  }
                }
              }
            }
            n75 = call <vilib>:"Add State(s) to Queue__jki_lib_state_machine.vi"("State(s) in (\"\")"=w222) -> ("States Out"=w221:string)  [unwired: 14 in]
          }
          frame "UI: Front Panel State" {
            # "Argument"
            # "Set Front Panel Open or Closed\n(Usage: \"UI: Front Panel State >> Open|Close\")"
            n76 = Unbundle By Name(w234) -> ("Core.Current VI Reference"=w233:refnum<vi>)
            n77 = disable-structure shown="Default" {
              disable-tunnel: w236 -> [w242 w265]
              disable-tunnel: [w241 w265] -> w235
              disable-tunnel: w233 -> [w240 _]
              disable-tunnel: w232 -> [w239 _]
              frame condition #0 (active) {
                n78 = case shown="\"Close\"" w239 {
                  tunnel: w242 -> [w246 w259]
                  tunnel: [w248 w260] -> w241
                  tunnel: w240 -> [w247 w257]
                  frame "Open", Default {
                    n79 = property class="VI"(reference=w247, error in=w246) -> (reference out=w244:refnum<vi>, error out=w245:errorcluster, "FP.State"=w243:T3)
                    n80 = case shown="\"Closed\"" w243 {
                      tunnel: [w251 w254] -> w248
                      tunnel: w245 -> [w250 w254]
                      tunnel: w244 -> [w249 _]
                      frame "Closed" {
                        n81 = invoke class="VI" method="FP.Open"(reference=w249, error in=w250, "Activate"=TRUE, "State"=T3."Standard") -> (error out=w251:errorcluster)  [unwired: 1 in, 4 out]
                      }
                      frame Default {
                      }
                    }
                  }
                  frame "Close" {
                    n82 = property class="VI"(reference=w257, error in=w259) -> (reference out=w256:refnum<vi>, error out=w258:errorcluster, "FP.State"=w255:T3)
                    n83 = case shown="Default" w255 {
                      tunnel: [w261 w264] -> w260
                      tunnel: w258 -> [w261 w263]
                      tunnel: w256 -> [_ w262]
                      frame "Invalid", "Closed" {
                      }
                      frame Default {
                        n84 = invoke class="VI" method="FP.Close"(reference=w262, error in=w263) -> (error out=w264:errorcluster)  [unwired: 1 in, 2 out]
                      }
                    }
                  }
                }
              }
              frame condition #1 {
              }
            }
            n85 = call <vilib>:"Add State(s) to Queue__jki_lib_state_machine.vi"("State(s) in (\"\")"=w238) -> ("States Out"=w237:string)  [unwired: 14 in]
          }
          frame "---------- Macro ----------" {
            # "Do not put any code in this frame.\n(It is a separator no-op. You can make a copy of this frame to create a new Macro frame)"
            n86 = call <vilib>:"Add State(s) to Queue__jki_lib_state_machine.vi"("State(s) in (\"\")"=w270) -> ("States Out"=w269:string)  [unwired: 14 in]
          }
          frame "Macro: Initialize" {
            w273 = "UI: Initialize\n//UI: Front Panel State >> Open"  # UI: Initialize //UI: Front Panel State >> Open
            # "Initialization Macro\n(This is called once, when the VI starts)"
            n87 = call <vilib>:"Add State(s) to Queue__jki_lib_state_machine.vi"("State(s) in Front (\"\")"="Data: Initialize\nInitialize Core Data\nEvents: Register", "State(s) in (\"\")"="Process: Sync", "State(s) at Back (\"\")"=w273) -> ("States Out"=w272:string)  [unwired: 12 in]
            n88 = call <vilib>:"Add State(s) to Queue__jki_lib_state_machine.vi"("State(s) in Front (\"\")"=w272, "State(s) in (\"\")"=w279) -> ("States Out"=w278:string)  [unwired: 13 in]
          }
          frame "Macro: Exit" {
            # "Exit Macro\n(This is called once, when the VI exits)"
            n89 = Unbundle By Name(w284) -> ("Core.Close Panel on Exit?"=w290:bool)
            n90 = Select(t="UI: Front Panel State >> Close", s=w290, f="") -> (s? t:f=w287:string)
            n91 = call <vilib>:"Add State(s) to Queue__jki_lib_state_machine.vi"("State(s) in Front (\"\")"="Data: Cleanup\nEvents: Unregister", "State(s) in (\"\")"="Process: Sync", "State(s) at Back (\"\")"="Exit") -> ("States Out"=w281:string)  [unwired: 12 in]
            n92 = call <vilib>:"Add State(s) to Queue__jki_lib_state_machine.vi"("State(s) in (\"\")"=w287, "State(s) at Back (\"\")"=w281) -> ("States Out"=w286:string)  [unwired: 13 in]
            n93 = call <vilib>:"Add State(s) to Queue__jki_lib_state_machine.vi"("State(s) in Front (\"\")"=w286, "State(s) in (\"\")"=w293) -> ("States Out"=w292:string)  [unwired: 13 in]
          }
          frame "---------- Process ----------" {
            # "Template Separator\n(You can make a copy of, or modify, this frame)"
            n94 = call <vilib>:"Add State(s) to Queue__jki_lib_state_machine.vi"("State(s) in (\"\")"=w298) -> ("States Out"=w297:string)  [unwired: 14 in]
          }
          frame "Process: Sync" {
            n95 = Unbundle By Name(w306) -> ("Self Reference"=w302:refnum<class "XYStage.KIM101.lvclass">)
            n96 = call <vilib>:"WaitOnProcessSync.vi"("error in (no error)"=w301, "SMO"=w302) -> ("error out"=w300:errorcluster, "Don't run?"=w305:bool)  [unwired: 7 in, 1 out]
            n97 = Select(t="Data: Cleanup\nEvents: Unregister\nExit", s=w305, f="") -> (s? t:f=w299:string)
            n98 = call <vilib>:"Add State(s) to Queue__jki_lib_state_machine.vi"("State(s) in Front (\"\")"=w299, "State(s) in (\"\")"=w309) -> ("States Out"=w308:string)  [unwired: 13 in]
          }
          frame "---------- Events ----------" {
            # "Template Separator\n(You can make a copy of, or modify, this frame)"
            n99 = call <vilib>:"Add State(s) to Queue__jki_lib_state_machine.vi"("State(s) in (\"\")"=w314) -> ("States Out"=w313:string)  [unwired: 14 in]
          }
          frame "Events: Register" {
            w325 = T15 {"Channel"=1, "IsEnabled"=FALSE, "IsError"=FALSE, "IsMoving"=FALSE, "Position"=0, "Status"=0}  # Inertial Motor Status
            # "XYStage.KIM101 Private Events"
            # "Create User Event for Callback"
            # "Device Public Events"
            n100 = Unbundle By Name(w323) -> ("Self Reference"=w334:refnum<class "XYStage.KIM101.lvclass">)
            n101 = call <vilib>:"GetProtectedEvents.vi"("SMO"=w334) -> ("error out"=w320:errorcluster, "SMO Protected Events"=w335:T16, "SMO out"=w327:refnum<class "XYStage.KIM101.lvclass">)  [unwired: 8 in]
            n102 = Create User Event(user event datatype=w325) -> (user event=w322:refnum<user-event>, error out=w319:errorcluster)  [unwired: 1 in]
            n103 = call "Device.GetPublicEventsRegistration.vi"("Device in"=w327) -> ("error out"=w326:errorcluster, "Device Public Events"=w328:refnum<event-registration>, "Device out"=w317:refnum<class "XYStage.KIM101.lvclass">)  [unwired: 8 in]
            n104 = call "XYStage.KIM101.GetPrivateEventsRegistration.vi"("XYStage.KIM101 in"=w317) -> ("error out"=w316:errorcluster, "XYStage.KIM101 Private Events"=w315:refnum<event-registration>)  [unwired: 8 in, 1 out]
            n105 = Bundle By Name(cluster=w323, "Status Update Event"=w322) -> (w321:T13)
            n106 = register-events(error in=w319, w322) -> (reference out=w324:refnum<event-registration>, error out=w318:errorcluster)  [unwired: 1 in]
            n107 = register-events(error in=w320, w335) -> (reference out=w330:refnum<event-registration>, error out=w332:errorcluster)  [unwired: 1 in]
            n108 = Bundle("Event Registration Refnum"=w330, "Device Public Events"=w328, "Event Registration Refnum"=w324, "XYStage.KIM101 Private Events"=w315) -> (w329:T17)  [unwired: 1 in]
            n109 = Merge Errors(w326, w333, w318, w332, w316) -> (w331:errorcluster)
            n110 = call <vilib>:"Add State(s) to Queue__jki_lib_state_machine.vi"("State(s) in (\"\")"=w337) -> ("States Out"=w336:string)  [unwired: 14 in]
          }
          frame "Events: Unregister" {
            n111 = Unregister For Events(event registration refnum=w340, error in=w339) -> (error out=w338:errorcluster)
            n112 = call <vilib>:"Clear Errors.vi"("error in (no error)"=w338) -> ()  [unwired: 5 in, 2 out]
            n113 = call <vilib>:"Add State(s) to Queue__jki_lib_state_machine.vi"("State(s) in (\"\")"=w343) -> ("States Out"=w342:string)  [unwired: 14 in]
          }
          frame "Events: Send OnStatusUpdate" {
            # "Send to Base XYStage class Process.vi"
            n114 = Unbundle By Name(w348) -> ("StatusUpdated"=w346:T10)
            n115 = call "XYStage.OnStatusUpdate.vi"("error in (no error)"=w345, "StatusUpdated"=w346, "XYStage"=w347) -> ("error out"=w344:errorcluster)  [unwired: 7 in, 1 out]
            n116 = call <vilib>:"Add State(s) to Queue__jki_lib_state_machine.vi"("State(s) in (\"\")"=w351) -> ("States Out"=w350:string)  [unwired: 14 in]
          }
          frame "Events: Send OnMoveResultReported" {
            w361 = T18 {"Result"=FALSE, "Coordinates"={"Units"={"X"=0.0, "Y"=0.0}, "Counts"={"X"=0, "Y"=0}}}  # MoveResultReported
            # "Send to Base XYStage class Process.vi"
            n117 = Unbundle By Name(w365) -> ("Current"=w360:T6, "Move Result.X axis need to move?"=w358:bool, "Move Result.X axis move result"=w357:bool, "Move Result.Y axis need to move?"=w356:bool, "Move Result.Y axis move result"=w355:bool)
            n118 = case shown="True" w358 {
              tunnel: w357 -> [_ w372]
              tunnel: [TRUE ("X axis move result") w372] -> w354
              frame False {
              }
              frame True {
              }
            }
            n119 = case shown="True" w356 {
              tunnel: w355 -> [_ w370]
              tunnel: [TRUE ("X axis move result") w370] -> w353
              frame False {
              }
              frame True {
              }
            }
            n120 = And(x=w354, y=w353) -> (x .and. y?=w352:bool)
            n121 = Bundle By Name(cluster=w361, "Result"=w352, "Coordinates"=w360) -> (w359:T18)
            n122 = call "XYStage.OnMoveResultReported.vi"("error in (no error)"=w363, "Move Result Reported"=w359, "XYStage"=w364) -> ("error out"=w362:errorcluster)  [unwired: 7 in, 1 out]
            n123 = call <vilib>:"Add State(s) to Queue__jki_lib_state_machine.vi"("State(s) in (\"\")"=w368) -> ("States Out"=w367:string)  [unwired: 14 in]
          }
          frame "---------- Action ----------" {
            n124 = call <vilib>:"Add State(s) to Queue__jki_lib_state_machine.vi"("State(s) in (\"\")"=w377) -> ("States Out"=w376:string)  [unwired: 14 in]
          }
          frame "Action: Subscribe for StatusUpdate Event" {
            n125 = Unbundle By Name(w382) -> ("Status Update Event"=w381:refnum<user-event>)
            n126 = call "XYStage.KIM101.GetResource.vi"("error in (no error)"=w380, "XYStage.KIM101 in"=w387) -> ("error out"=w379:errorcluster, "Resource"=w386:T19)  [unwired: 7 in, 1 out]
            n127 = Unbundle By Name(w386) -> ("Device"=w385:refnum<k24>)
            n128 = vi-ref "XYStage.KIM101.lvclass:StatusUpdate Callback.vi"() -> (w384:refnum<vi>)
            n129 = node(w379, w385, w384, w381) -> (w378:errorcluster)  [unwired: 1 in, 1 out]
            n130 = call <vilib>:"Add State(s) to Queue__jki_lib_state_machine.vi"("State(s) in (\"\")"=w389) -> ("States Out"=w388:string)  [unwired: 14 in]
          }
          frame "Action: Move Absolute (counts)" {
            w394 = "\r\n"
            # "TODO: Control Timeouts"
            n131 = Unbundle By Name(w392) -> ("Target.Counts.X"=w403:i32, "Current.Counts.X"=w402:i32)
            n132 = Unbundle By Name(w392) -> ("Target.Counts.Y"=w400:i32, "Current.Counts.Y"=w399:i32)
            n133 = Not Equal?(x=w403, y=w402) -> (x != y?=w401:bool)
            n134 = Not Equal?(x=w400, y=w399) -> (x != y?=w398:bool)
            n135 = case shown="False" w401 {
              tunnel: [_ "Action: Move Absolute By Axis (counts) >> X Axis\nAction: Wait for Move Complete (counts) >> X Axis\nAction: Set Wait Result By Axis >> X Axis"] -> w397
              tunnel: w392 -> [w417 w420]
              tunnel: [w415 w418] -> w391
              frame False {
                n136 = Bundle By Name(cluster=w417, "Move Result.X axis need to move?"=FALSE) -> (w415:T13)
              }
              frame True {
                n137 = Bundle By Name(cluster=w420, "Move Result.X axis need to move?"=TRUE) -> (w418:T13)
              }
            }
            n138 = case shown="True" w398 {
              tunnel: [_ "Action: Move Absolute By Axis (counts) >> Y Axis\nAction: Wait for Move Complete (counts) >> Y Axis\nAction: Set Wait Result By Axis >> Y Axis"] -> w395
              tunnel: w391 -> [w410 w413]
              tunnel: [w408 w411] -> w390
              frame False {
                n139 = Bundle By Name(cluster=w410, "Move Result.Y axis need to move?"=FALSE) -> (w408:T13)
              }
              frame True {
                n140 = Bundle By Name(cluster=w413, "Move Result.Y axis need to move?"=TRUE) -> (w411:T13)
              }
            }
            n141 = Concatenate Strings(w397, w394, w395, w394, "Events: Send OnMoveResultReported" ("string")) -> (w396:string)
            n142 = call <vilib>:"Add State(s) to Queue__jki_lib_state_machine.vi"("State(s) in Front (\"\")"=w396, "State(s) in (\"\")"=w407) -> ("States Out"=w406:string)  [unwired: 13 in]
          }
          frame "Action: Move Absolute By Axis (counts)" {
            n143 = case shown="\"X Axis\"" w425 {
              tunnel: w424 -> [w434 _ w437]
              tunnel: [XYStage.Axis--Enum."Y Axis" ("Axis") _ XYStage.Axis--Enum."X Axis" ("Axis")] -> w423
              tunnel: [w432 _ w435] -> w422
              frame "Y Axis" {
                n144 = Unbundle By Name(w434) -> ("Target.Counts.Y"=w432:i32)
              }
              frame "", Default {
              }
              frame "X Axis" {
                n145 = Unbundle By Name(w437) -> ("Target.Counts.X"=w435:i32)
              }
            }
            n146 = call "XYStage.KIM101.MoveAbsoluteByAxis (counts).vi"("error in (no error)"=w427, "Position (counts)"=w422, "Axis"=w423, "XYStage.KIM101 in"=w428) -> ("error out"=w426:errorcluster)  [unwired: 6 in, 1 out]
            n147 = call <vilib>:"Add State(s) to Queue__jki_lib_state_machine.vi"("State(s) in (\"\")"=w431) -> ("States Out"=w430:string)  [unwired: 14 in]
          }
          frame "Action: Wait for Move Complete (counts)" {
            n148 = case shown="\"X Axis\"" w444 {
              tunnel: w443 -> [w450 _ w453]
              tunnel: [XYStage.Axis--Enum."Y Axis" ("Axis") _ XYStage.Axis--Enum."X Axis" ("Axis")] -> w440
              tunnel: [w448 _ w451] -> w439
              frame "Y Axis" {
                n149 = Unbundle By Name(w450) -> ("Target.Counts.Y"=w448:i32)
              }
              frame "", Default {
              }
              frame "X Axis" {
                n150 = Unbundle By Name(w453) -> ("Target.Counts.X"=w451:i32)
              }
            }
            n151 = Bundle By Name(cluster=w443, "Wait.In Wait?"=TRUE ("In Wait?"), "Wait.Axis"=w440, "Wait.Position"=w439, "Wait.Next Steps"=w438) -> (w442:T13)
            n152 = call <vilib>:"Add State(s) to Queue__jki_lib_state_machine.vi"() -> ("States Out"=w447:string)  [unwired: 15 in]
          }
          frame "Action: Wait Processor" {
            n153 = Unbundle By Name(w457) -> ("StatusUpdated.Axis"=w459:T4, "StatusUpdated.Position"=w458:i32)
            n154 = Unbundle By Name(w457) -> ("Wait.Axis"=w462:T4, "Wait.Position"=w461:i32, "Wait.Next Steps"=w460:string)
            n155 = Equal?(x=w462, y=w459) -> (x = y?=w454:bool)
            n156 = case shown="True" w454 {
              tunnel: w458 -> [_ w473]
              tunnel: w461 -> [_ w474]
              tunnel: w460 -> [_ w471]
              tunnel: [_ w470] -> w455
              tunnel: w457 -> [w467 w469]
              tunnel: [w467 w468] -> w456
              frame False {
              }
              frame True {
                n157 = Equal?(x=w474, y=w473) -> (x = y?=w472:bool)
                n158 = case shown="True" w472 {
                  tunnel: w471 -> [_ w477]
                  tunnel: [_ w477] -> w470
                  tunnel: w469 -> [w475 w480]
                  tunnel: [w475 w478] -> w468
                  frame False {
                  }
                  frame True {
                    n159 = Bundle By Name(cluster=w480, "Wait.In Wait?"=FALSE ("In Wait?"), "Wait.Result"=TRUE ("WaitResult")) -> (w478:T13)
                  }
                }
              }
            }
            n160 = call <vilib>:"Add State(s) to Queue__jki_lib_state_machine.vi"("State(s) in Front (\"\")"=w455, "State(s) in (\"\")"=w466) -> ("States Out"=w465:string)  [unwired: 13 in]
          }
          frame "Action: Set Wait Result By Axis" {
            n161 = Unbundle By Name(w482) -> ("Wait.Result"=w483:bool)
            n162 = case shown="\"X Axis\"" w484 {
              tunnel: w483 -> [w491 _ w494]
              tunnel: w482 -> [w490 w492 w495]
              tunnel: [w489 w492 w493] -> w481
              frame "Y Axis" {
                n163 = Bundle By Name(cluster=w490, "Move Result.Y axis move result"=w491) -> (w489:T13)
              }
              frame "", Default {
              }
              frame "X Axis" {
                n164 = Bundle By Name(cluster=w495, "Move Result.X axis move result"=w494) -> (w493:T13)
              }
            }
            n165 = call <vilib>:"Add State(s) to Queue__jki_lib_state_machine.vi"("State(s) in (\"\")"=w488) -> ("States Out"=w487:string)  [unwired: 14 in]
          }
        }
      }
    }
    frame Error {
    }
  }
  n166 = call-parent "Process.vi"("error in"=w8, "XYStage"=w7) -> ("error out"=w5:errorcluster, "XYStage out"=→"XYStage.KIM101 out":refnum<class "XYStage.KIM101.lvclass">)  [unwired: 8 in]
  n167 = Merge Errors(w5, w4) -> (→"error out":errorcluster)
